vi "serial_init.vi"() -> (0 "error out":errorcluster, 2 "Cancelled?":bool, 3 "VISA out":refnum<visa-resource-name>)   [LabVIEW 2023]
uses:
  <vilib>/Instr/_visa.llb/VISA Configure Serial Port (Instr).vi
panel:
  in  "cancel":bool
  in  "ok":bool
  in  "COM port":refnum<visa-resource-name>
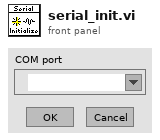
[diagram p1: front panel]
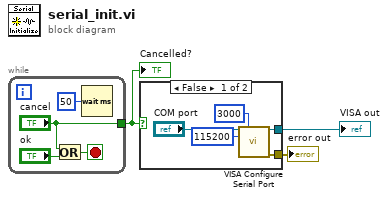
[diagram p0: block diagram]
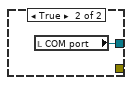
[diagram p2: hidden frame]
diagram:
  n1 = while {
    tunnel: ["cancel"] -> w3
    stop <- w5 stop-if-true
    n2 = Or(x="cancel", y="ok") -> (x .or. y?=w5:bool)
    n3 = Wait (ms)(milliseconds to wait=u32 50) -> ()  [unwired: 1 out]
  }
  "Cancelled?" <- w3
  n4 = case shown="False" w3 {
    tunnel: [w9 w13] -> w2
    tunnel: [w8 _] -> w1
    frame False {
      n5 = call-poly "VISA Configure Serial Port"("VISA resource name"="COM port", "timeout (10sec)"=u32 3000, "baud rate (9600)"=u32 115200) -> ("VISA resource name out"=w9:refnum<visa-resource-name>, "error out"=w8:errorcluster)  [unwired: 11 in]
    }
    frame True {
      n6 = local read "COM port"() -> (w13:refnum<visa-resource-name>)
    }
  }
  "VISA out" <- w2
  "error out" <- w1
